vi "PBLV_Example_SOS-Loop.vi"() -> ()   [LabVIEW 2010]
panel:
  in  "Array":T1(array[cluster])=[{"Instruct Data"=3, "Op Code"=2, "Flags"=[TRUE, FALSE, FALSE, FALSE, FALSE, FALSE, FALSE, FALSE, FALSE, FALSE, FALSE, FALSE, FALSE, FALSE, FALSE, FALSE, FALSE, FALSE, FALSE, FALSE, FALSE, FALSE, FALSE, FALSE], "Comments"="S                 . . .", "Time (s)"=0.1}, {"Instruct Data"=0, "Op Code"=3, "Flags"=[FALSE, FALSE, FALSE, FALSE, FALSE, FALSE, FALSE, FALSE, FALSE, FALSE, FALSE, FALSE, FALSE, FALSE, FALSE, FALSE, FALSE, FALSE, FALSE, FALSE, FALSE, FALSE, FALSE, FALSE], "Comments"="", "Time (s)"=0.1}, {"Instruct Data"=3, "Op Code"=2, "Flags"=[TRUE, FALSE, FALSE, FALSE, FALSE, FALSE, FALSE, FALSE, FALSE, FALSE, FALSE, FALSE, FALSE, FALSE, FALSE, FALSE, FALSE, FALSE, FALSE, FALSE, FALSE, FALSE, FALSE, FALSE], "Comments"="O              - - -", "Time (s)"=0.3}, {"Instruct Data"=2, "Op Code"=3, "Flags"=[FALSE, FALSE, FALSE, FALSE, FALSE, FALSE, FALSE, FALSE, FALSE, FALSE, FALSE, FALSE, FALSE, FALSE, FALSE, FALSE, FALSE, FALSE, FALSE, FALSE, FALSE, FALSE, FALSE, FALSE], "Comments"="", "Time (s)"=0.1}, {"Instruct Data"=3, "Op Code"=2, "Flags"=[TRUE, FALSE, FALSE, FALSE, FALSE, FALSE, FALSE, FALSE, FALSE, FALSE, FALSE, FALSE, FALSE, FALSE, FALSE, FALSE, FALSE, FALSE, FALSE, FALSE, FALSE, FALSE, FALSE, FALSE], "Comments"="S                 . . .", "Time (s)"=0.1}, {"Instruct Data"=4, "Op Code"=3, "Flags"=[FALSE, FALSE, FALSE, FALSE, FALSE, FALSE, FALSE, FALSE, FALSE, FALSE, FALSE, FALSE, FALSE, FALSE, FALSE, FALSE, FALSE, FALSE, FALSE, FALSE, FALSE, FALSE, FALSE, FALSE], "Comments"="", "Time (s)"=0.1}, {"Instruct Data"=0, "Op Code"=6, "Flags"=[FALSE, FALSE, FALSE, FALSE, FALSE, FALSE, FALSE, FALSE, FALSE, FALSE, FALSE, FALSE, FALSE, FALSE, FALSE, FALSE, FALSE, FALSE, FALSE, FALSE, FALSE, FALSE, FALSE, FALSE], "Comments"="", "Time (s)"=0.5}] {"Time (s)" format="%.3p"; "Op Code" items=["Continue", "Stop", "Loop", "End Loop", "JSR", "RTS", "Branch", "Long Delay", "Wait"]}
  in  "Path to spinapi.dll":path=path "C:/SpinCore/SpinAPI/dll/spinapi.dll"
  in  "start/restart":bool
  in  "load":bool
  in  "stop":bool
  in  "clock_freq (MHz)":dbl=100.0
  # "LabVIEW PulseBlaster Extension\nSOS-Loop\nSpinCore Technologies, Inc.\nwww.spincore.com"
  # "Inst 0"
  # "Inst 1"
  # "Inst 2"
  # "Inst 3"
  # "Inst 4"
  # "Inst 5"
  # "Inst 6"
  # "Caution:    \n            After pressing \n            STOP, all output bits may maintain their final state."
  # "1"
  # "2"
  # "3"
  # "4"
  # "5"
  # "6"
  # "7"
  # "8"
  # "9"
  # "10"
  # "11"
  # "12"
  # "13"
  # "14"
  # "15"
  # "16"
  # "17"
  # "18"
  # "19"
  # "20"
  # "21"
  # "22"
  # "23"
  # "24"
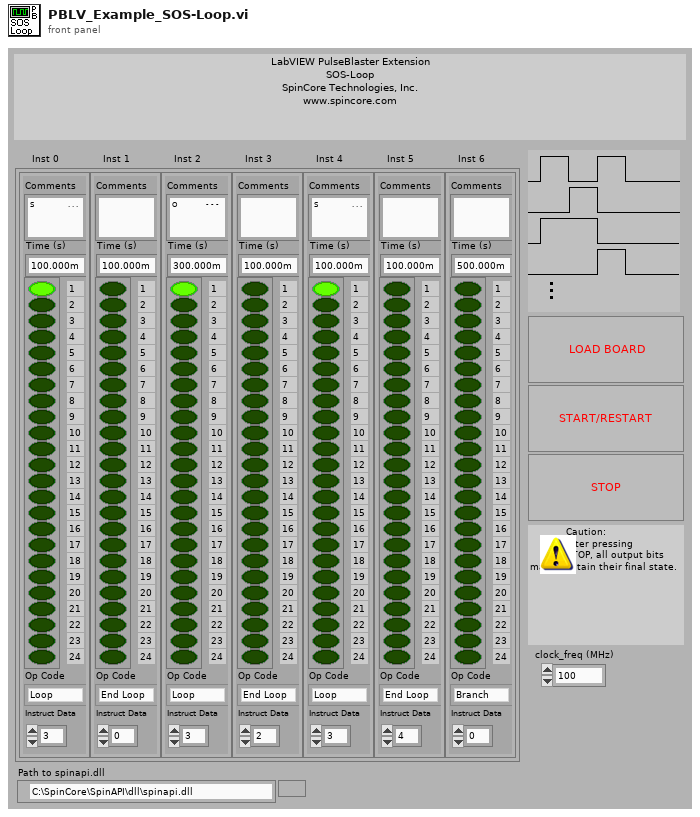
[diagram p1: front panel]
types:
  T1 = cluster{"Instruct Data":i32, "Op Code":i32, "Flags":bool[], "Comments":string, "Time (s)":dbl}[]
  T2 = enum16{"Pulse Program", "Frequency Registers", "TX Phase Registers", "RX Phase Registers"}
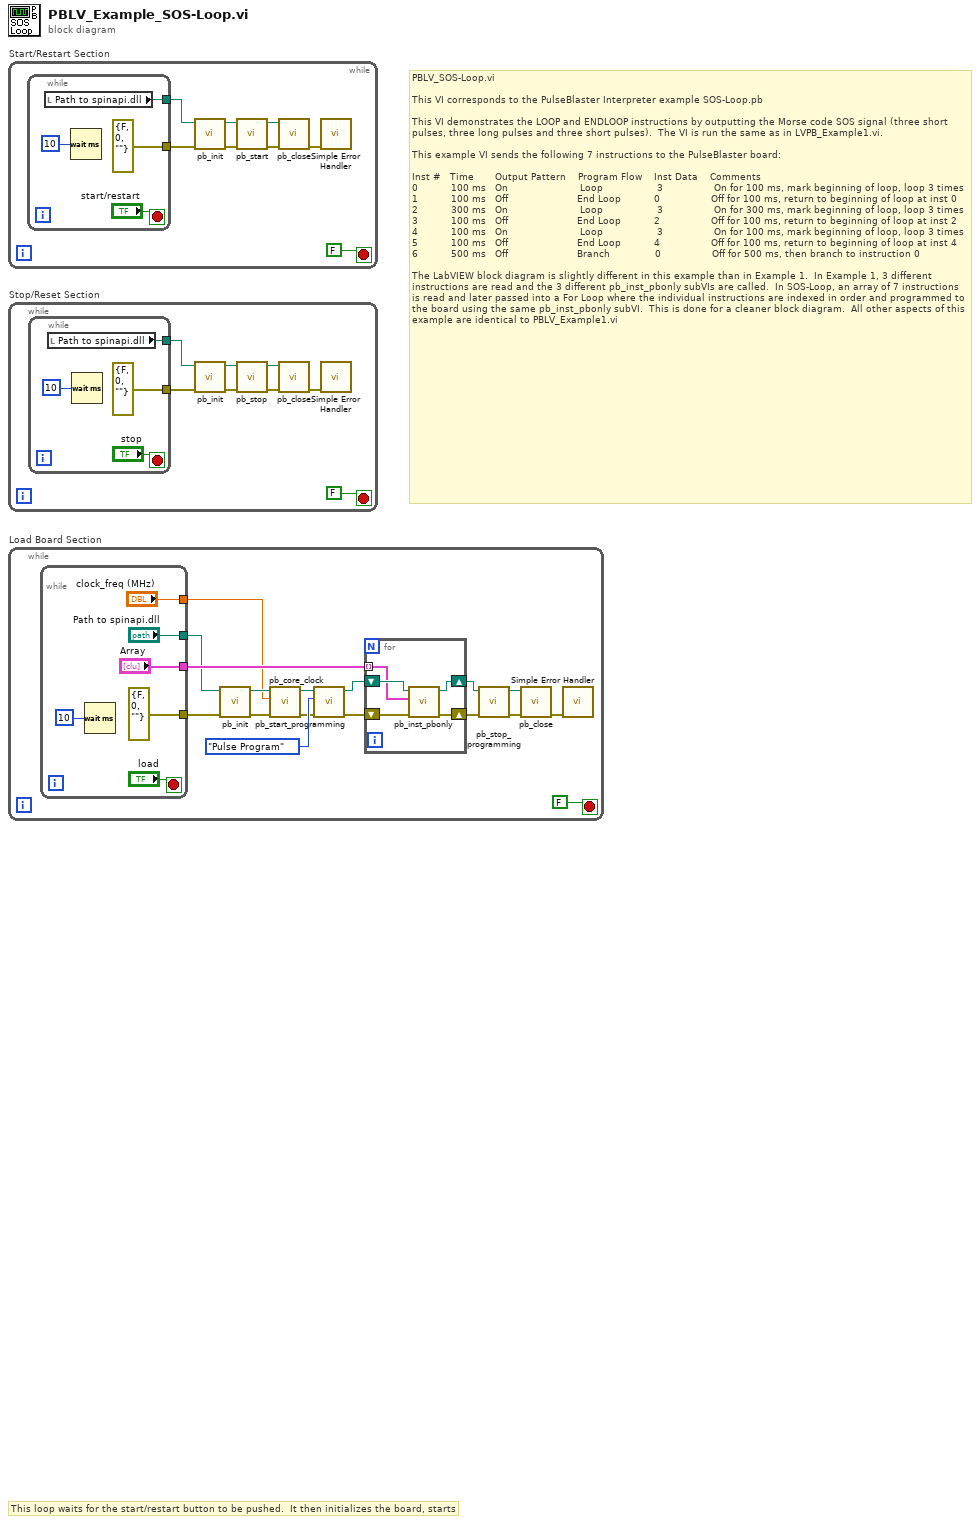
[diagram p0: block diagram]
diagram:
  # "PBLV_SOS-Loop.vi\n\nThis VI corresponds to the PulseBlaster Interpreter example SOS-Loop.pb\n\nThis VI demonstrates the LOOP and ENDLOOP instructions by outputting the Morse code SOS signal (three short pulses, three long pulses and three short pulses).  The VI is run the same as in LVPB_Example1.vi. \n\nThis example VI sends the following 7 instructions to the PulseBlaster board:\n\nInst #   Time       Output Pattern    Program Flow    Inst Data    Comments\n0           100 ms   On                        Loop                  3                 On for 100 ms, mark beginning of loop, loop 3 times\n1           100 ms   Off                       End Loop           0                 Off for 100 ms, return to beginning of loop at inst 0\n2           300 ms   On                        Loop                  3                 On for 300 ms, mark beginning of loop, loop 3 times \n3           100 ms   Off                       End Loop           2                 Off for 100 ms, return to beginning of loop at inst 2\n4           100 ms   On                        Loop                  3                 On for 100 ms, mark beginning of loop, loop 3 times\n5           100 ms   Off                       End Loop           4                 Off for 100 ms, return to beginning of loop at inst 4\n6           500 ms   Off                       Branch               0                 Off for 500 ms, then branch to instruction 0\n\nThe LabVIEW block diagram is slightly different in this example than in Example 1.  In Example 1, 3 different instructions are read and the 3 different pb_inst_pbonly subVIs are called.  In SOS-Loop, an array of 7 instructions is read and later passed into a For Loop where the individual instructions are indexed in order and programmed to the board using the same pb_inst_pbonly subVI.  This is done for a cleaner block diagram.  All other aspects of this example are identical to PBLV_Example1.vi"
  # "This loop waits for the start/restart button to be pushed.  It then initializes the board, starts"
  n1 = while "Start/Restart Section" {
    stop <- FALSE stop-if-true
    n2 = while {
      tunnel: [errorcluster {"status"=FALSE, "code"=0, "source"=""} ("error in (no error)")] -> w5
      tunnel: [w9] -> w1
      stop <- "start/restart" stop-if-true
      n3 = local read "Path to spinapi.dll"() -> (w9:path)
      n4 = Wait (ms)(milliseconds to wait=u32 10) -> ()  [unwired: 1 out]
    }
    n5 = call "pb_init.vi"("error in (no error)"=w5, "path in"=w1) -> ("error out"=w4:errorcluster, "path out"=w7:path)  [unwired: 1 in, 7 out]
    n6 = call "pb_start.vi"("error in (no error)"=w4, "path in"=w7) -> ("error out"=w3:errorcluster, "path out"=w8:path)  [unwired: 1 in, 7 out]
    n7 = call "pb_close.vi"("error in (no error)"=w3, "path in"=w8) -> ("error out"=w2:errorcluster)  [unwired: 9 out]
    n8 = call <vilib>:"Simple Error Handler.vi"("error in (no error)"=w2) -> ()  [unwired: 1 in, 8 out]
  }
  n9 = while "Stop/Reset Section" {
    stop <- FALSE stop-if-true
    n10 = while {
      tunnel: [errorcluster {"status"=FALSE, "code"=0, "source"=""} ("error in (no error)")] -> w17
      tunnel: [w21] -> w13
      stop <- "stop" stop-if-true
      n11 = local read "Path to spinapi.dll"() -> (w21:path)
      n12 = Wait (ms)(milliseconds to wait=u32 10) -> ()  [unwired: 1 out]
    }
    n13 = call "pb_init.vi"("error in (no error)"=w17, "path in"=w13) -> ("error out"=w16:errorcluster, "path out"=w19:path)  [unwired: 1 in, 7 out]
    n14 = call "pb_stop.vi"("error in (no error)"=w16, "path in"=w19) -> ("error out"=w15:errorcluster, "path out"=w20:path)  [unwired: 8 out]
    n15 = call "pb_close.vi"("error in (no error)"=w15, "path in"=w20) -> ("error out"=w14:errorcluster)  [unwired: 9 out]
    n16 = call <vilib>:"Simple Error Handler.vi"("error in (no error)"=w14) -> ()  [unwired: 1 in, 8 out]
  }
  n17 = while "Load Board Section" {
    stop <- FALSE stop-if-true
    n18 = while {
      tunnel: [errorcluster {"status"=FALSE, "code"=0, "source"=""} ("error in (no error)")] -> w37
      tunnel: ["Array"] -> w31
      tunnel: ["Path to spinapi.dll"] -> w26
      tunnel: ["clock_freq (MHz)"] -> w25
      stop <- "load" stop-if-true
      n19 = Wait (ms)(milliseconds to wait=u32 10) -> ()  [unwired: 1 out]
    }
    n20 = call "pb_init.vi"("error in (no error)"=w37, "path in"=w26) -> ("error out"=w28:errorcluster, "path out"=w30:path)  [unwired: 2 in, 6 out]
    n21 = call "pb_core_clock.vi"("error in (no error)"=w28, "clock_freq (MHz)"=w25, "path in"=w30) -> ("error out"=w27:errorcluster, "path out"=w29:path)  [unwired: 7 in]
    n22 = call "pb_start_programming.vi"("error in (no error)"=w27, "Device"=T2."Pulse Program", "path in"=w29) -> ("error out"=w35:errorcluster, "path out"=w41:path)  [unwired: 1 in, 6 out]
    n23 = for {
      shift-right: [w45] -> w38
      shift-left: w41 -> [w46]
      shift-right: [w43] -> w34
      shift-left: w35 -> [w44]
      tunnel: w31 -> [w42] mode=indexing
      n24 = call "pb_inst_pbonly.vi"("error in (no error)"=w44, "PB Instruction"=w42, "path in"=w46) -> ("error out"=w43:errorcluster, "path out"=w45:path)  [unwired: 2 in, 5 out]
    }
    n25 = call "pb_stop_programming.vi"("error in (no error)"=w34, "path in"=w38) -> ("error out"=w33:errorcluster, "path out"=w40:path)  [unwired: 1 in, 7 out]
    n26 = call "pb_close.vi"("error in (no error)"=w33, "path in"=w40) -> ("error out"=w32:errorcluster)  [unwired: 9 out]
    n27 = call <vilib>:"Simple Error Handler.vi"("error in (no error)"=w32) -> ()  [unwired: 1 in, 8 out]
  }
